vi "XIPIN_AXI_Protocol_Checker_1_1.vi"   [LabVIEW 2017]
doc: "The AXI Protocol Checker.\n------------------------------------\n<b>Need License</b> : No\n<b>Interface</b> : AXI4"
uses:
  <vilib>/rvi/XilinxIP/XIPIN_XNode/niFpgaXIPIN.xnode
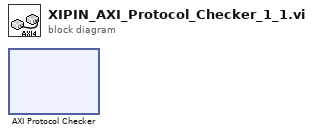
[diagram p0: block diagram]
diagram:
  n1 = xnode ("AXI Protocol Checker")() -> ()
